vi "Apply Softlimit.vi"(8 "error in (no error)":errorcluster, 11 "Motor in":refnum<class "Motor.lvclass">) -> (0 "error out":errorcluster, 3 "Motor out":refnum<class "Motor.lvclass">)   [LabVIEW 2016, in "Hardware.lvlib" / "Motor.lvlib" / "Motor.lvclass"]
uses:
  <userlib>/Common Components/Hardware/Motor/Motor/Motor.lvclass
  <userlib>/Common Components/Hardware/Motor/Motor/Motor.lvclass/Motor.ctl
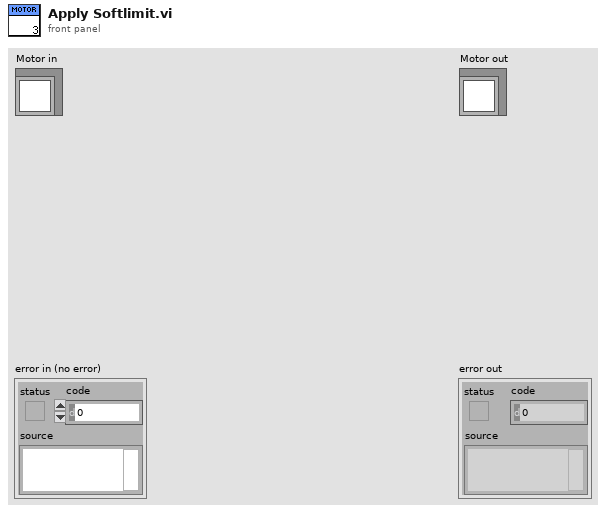
[diagram p1: front panel]
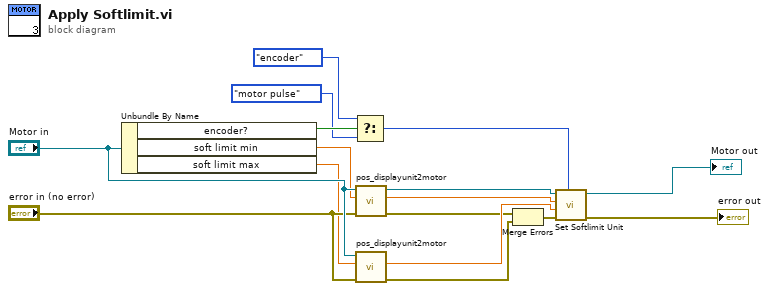
[diagram p0: block diagram]
diagram:
  n1 = Unbundle By Name("Motor in") -> ("encoder?"=w14:bool, "soft limit min"=w2:dbl, "soft limit max"=w1:dbl)
  n2 = Select(t=enum16{"motor pulse", "encoder"}."encoder" ("source_sel"), s=w14, f=enum16{"motor pulse", "encoder"}."motor pulse" ("source_sel")) -> (s? t:f=w13:enum16{"motor pulse", "encoder"})
  n3 = call <userlib>:"pos_displayunit2motor.vi"("error in (no error)"="error in (no error)", "pos in display unit"=w2, "Motor in"="Motor in") -> ("error out"=w6:errorcluster, "pos in motor (pulses)"=w9:dbl, "Motor out"=w3:refnum<class "Motor.lvclass">)  [unwired: 6 in]
  n4 = call <userlib>:"pos_displayunit2motor.vi"("error in (no error)"="error in (no error)", "pos in display unit"=w1, "Motor in"="Motor in") -> ("error out"=w5:errorcluster, "pos in motor (pulses)"=w8:dbl)  [unwired: 6 in, 1 out]
  n5 = Merge Errors(w6, w5) -> (w4:errorcluster)
  n6 = call-dynamic "Set Softlimit Unit.vi"("source_sel"=w13, "error in (no error)"=w4, "P_limit"=w8, "N_limit"=w9, "Motor in"=w3) -> ("error out"=→"error out":errorcluster, "Motor out"=→"Motor out":refnum<class "Motor.lvclass">)  [unwired: 5 in]
